vi "24Bitto18Bit.vi"(11 "24-Bit":u32=16 format="%024b") -> (3 "18Bit":u32)   [LabVIEW 2013]
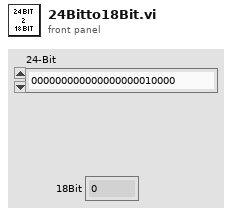
[diagram p1: front panel]
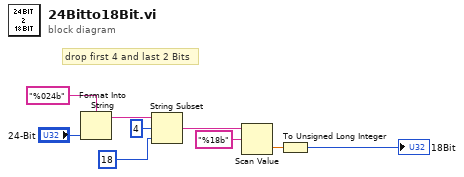
[diagram p0: block diagram]
diagram:
  # "drop first 4 and last 2 Bits"
  n1 = Format Into String(format string="%024b", "24-Bit") -> (resulting string=w7:string)  [unwired: 2 in, 1 out]
  n2 = String Subset(string=w7, offset (0)=4, length (rest)=18 ("length (rest)")) -> (substring=w4:string)
  n3 = Scan Value(string=w4, format string="%18b") -> (value=w2:dbl)  [unwired: 1 in, 1 out]
  n4 = To Unsigned Long Integer(number=w2) -> (unsigned 32bit integer=→"18Bit":u32)
